vi "Channel Get Modbus Type.vi"(8 "error in (no error)":errorcluster, 11 "Channel Ref":T1 format="%.0x") -> (0 "error out":errorcluster, 1 "Is MB Type?":bool, 2 "Type":T2, 3 "Item Ref out":T1 format="%.0x")   [LabVIEW 2020, in "Modbus Master System Explorer.lvlib"]
uses:
  Modbus Master System Explorer.lvlib
  <vilib>/NI VeriStand/Custom Device API/Custom Device Item Ref.ctl
  Modbus Type.ctl
  Shared/Constants.vi
  <vilib>/NI VeriStand/Custom Device API/Get Item Property (U16).vi
  Shared/Modbus Master Shared.lvlib
  <vilib>/NI VeriStand/Custom Device API/Custom Device API.lvlib
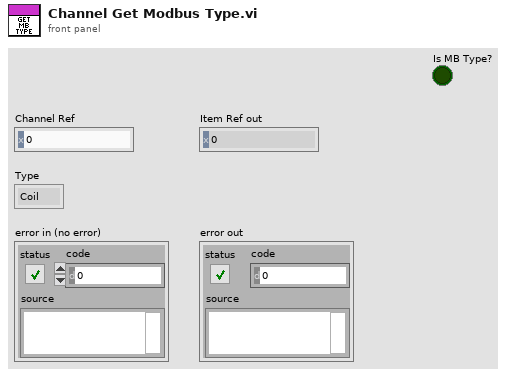
[diagram p1: front panel]
types:
  T1 = typedef "Custom Device API.lvlib/Custom Device Item Ref.ctl" = u64
  T2 = typedef "Modbus Master Shared.lvlib/Modbus Type.ctl" = enum16{"Coil", "Discrete Input", "Holding Register", "Input Register"}
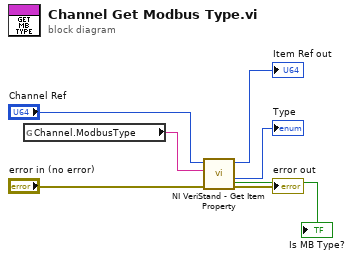
[diagram p0: block diagram]
diagram:
  n1 = global read "Constants.vi" "Channel.ModbusType"() -> (w3:string)
  n2 = call-poly <vilib>:"NI VeriStand - Get Item Property.vi"("error in (no error)"="error in (no error)", "Property Name"=w3, "Item Ref in"="Channel Ref") -> ("error out"=→"error out":errorcluster, "Value"=→"Type":u16, "Item Ref out"=→"Item Ref out":T1, "Found?"=→"Is MB Type?":bool)  [unwired: 5 in]
